vi "Dual_DM_Control_Main_V4.vi"() -> ()   [LabVIEW 2014]
uses:
  Controls/MirrorModes.ctl
  Controls/Standard Action.ctl
  <vilib>/Analysis/baseanly.llb/Mean (DBL).vi
  <vilib>/Utility/file.llb/Write To Spreadsheet File (DBL).vi
  <vilib>/Utility/file.llb/Read From Spreadsheet File (DBL).vi
  <vilib>/Analysis/NI_AALBase.lvlib
panel:
  in  "Active Mirror":enum32{"Mirror 1", "Mirror 2"}(radio)
  in  "Clear Modes":bool
  in  "Mirror Modes":T1
  in  "Load Modes":bool
  in  "Save Modes":bool
  in  "Scan Modes":bool
  in  "Load Flat":bool
  in  "Apply Zero":bool
  in  "Load V Map":bool
  in  "Save V Map":bool
  in  "Apply Flat":bool
  in  "Center Bias":bool
  in  "Exit":bool
  out "Pixel Map (-1 to 1)":dbl[][](graph)
  # "Mode"
  # "Amount (nm)"
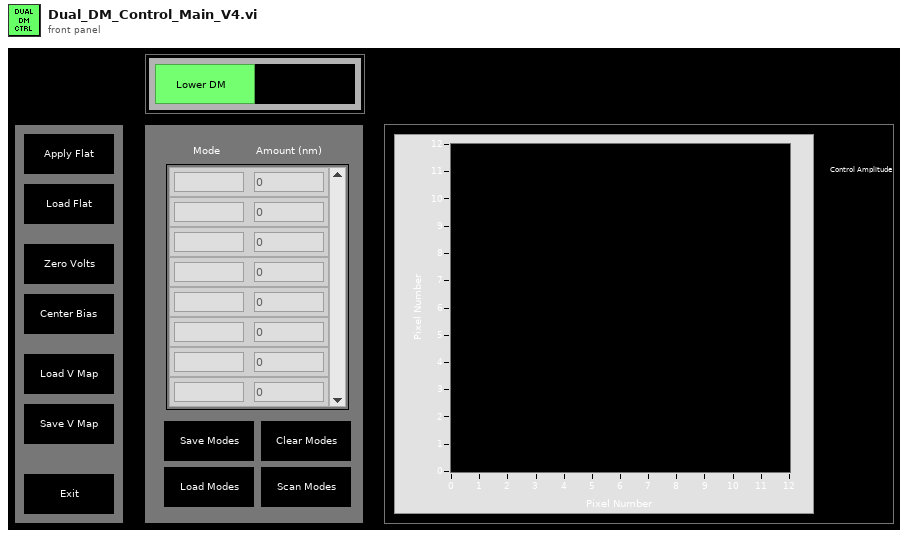
[diagram p1: front panel]
types:
  T1 = typedef "MirrorModes.ctl" = cluster{"Mode":string, "Amplitude":dbl}[]
  T2 = typedef "Standard Action.ctl" = enum16{"Read", "Write"}
  T3 = typedef "MirrorModes_DUAL.ctl" = cluster{"Mode":string, "Amplitude":dbl}[][]
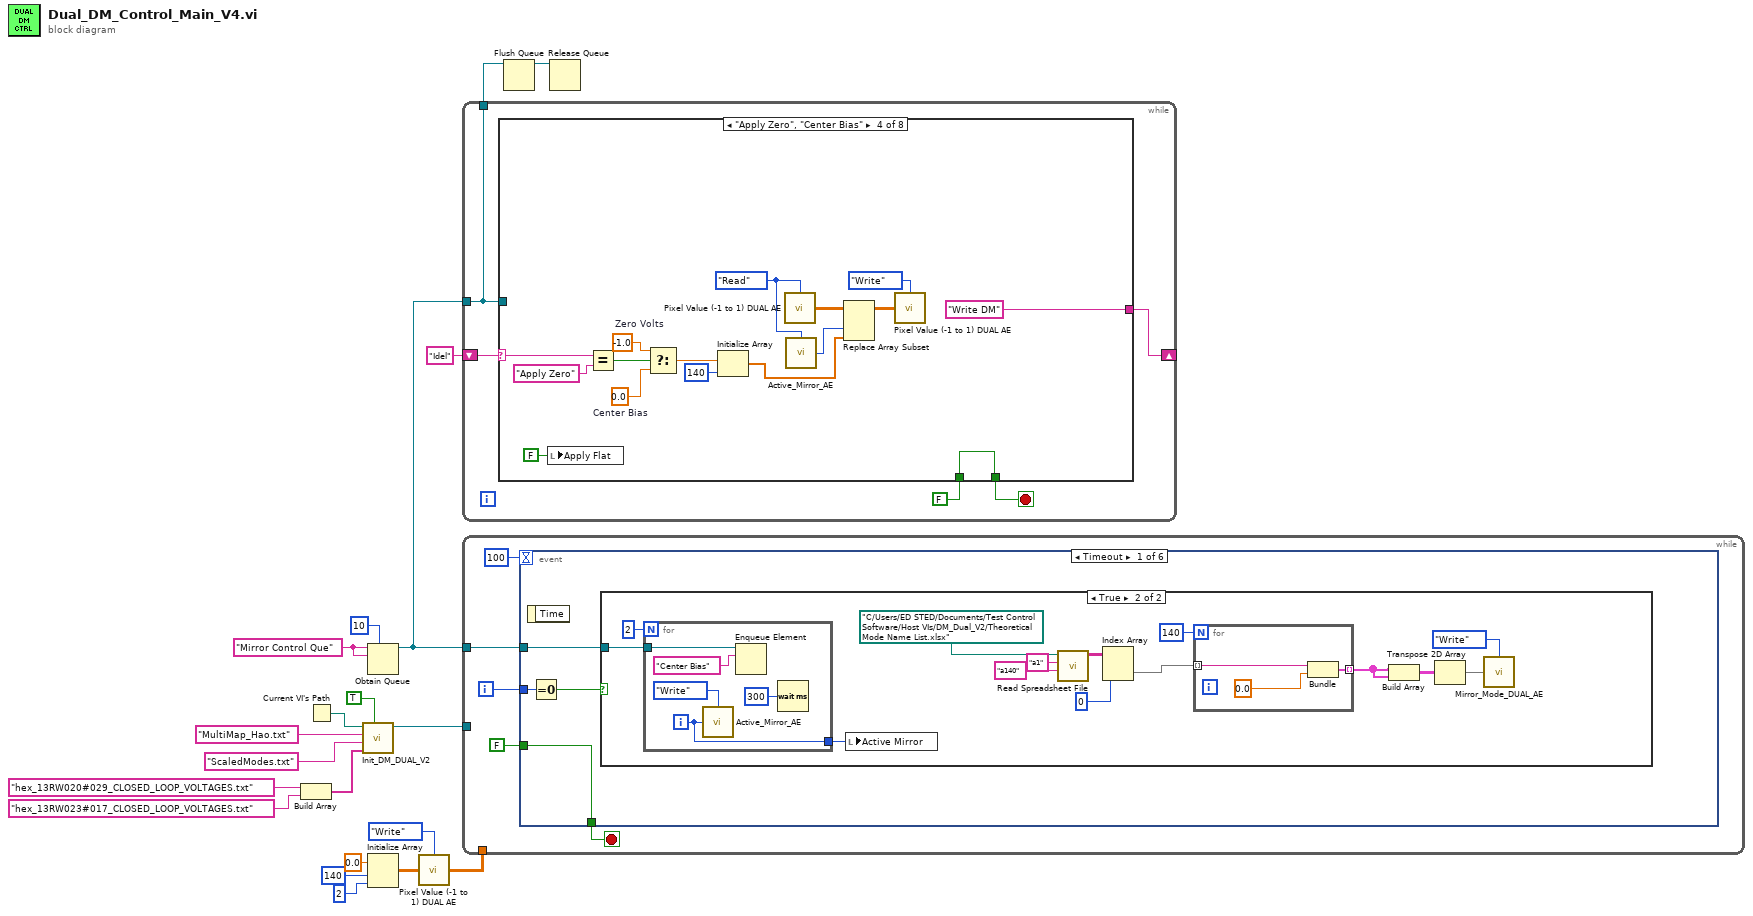
[diagram p0: block diagram]
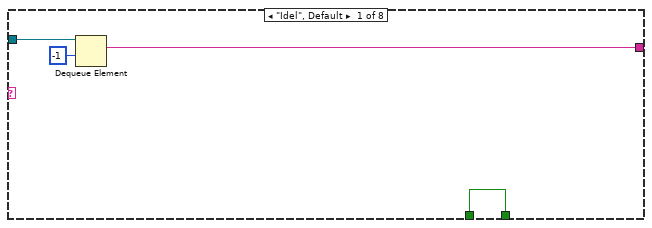
[diagram p2: hidden frame]
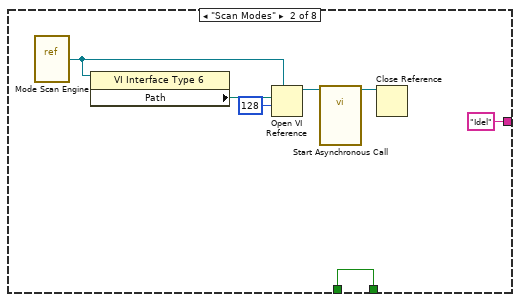
[diagram p3: hidden frame]
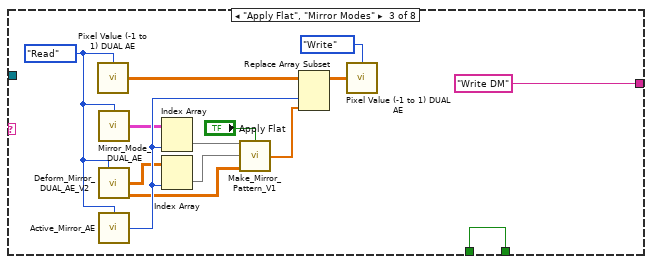
[diagram p4: hidden frame]
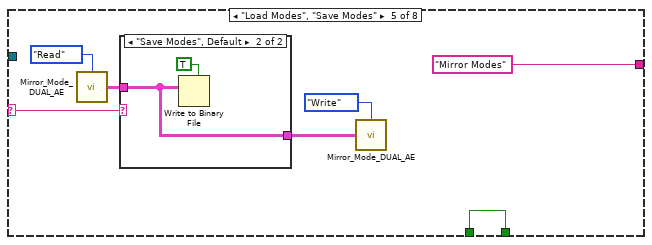
[diagram p5: hidden frame]
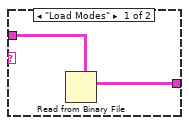
[diagram p6: hidden frame]
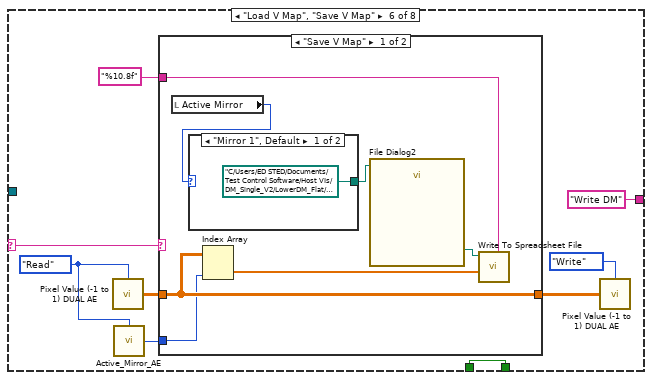
[diagram p7: hidden frame]
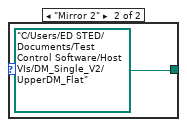
[diagram p8: hidden frame]
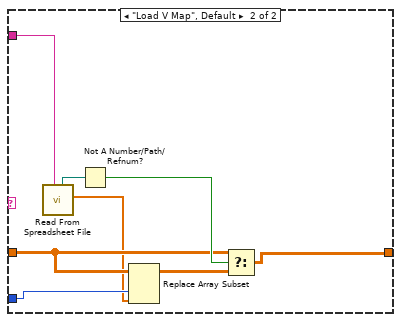
[diagram p9: hidden frame]
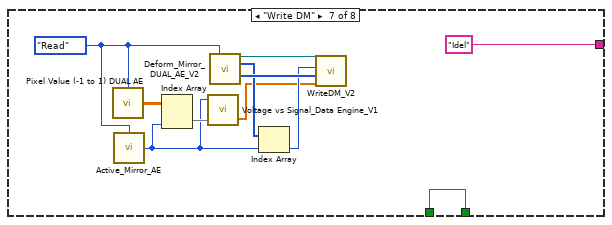
[diagram p10: hidden frame]
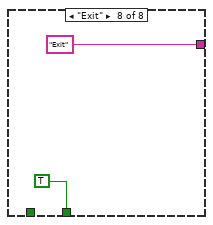
[diagram p11: hidden frame]
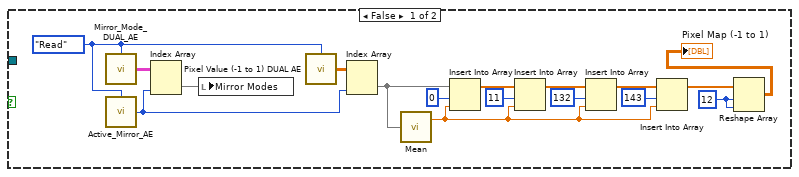
[diagram p12: hidden frame]
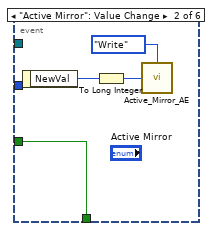
[diagram p13: hidden frame]
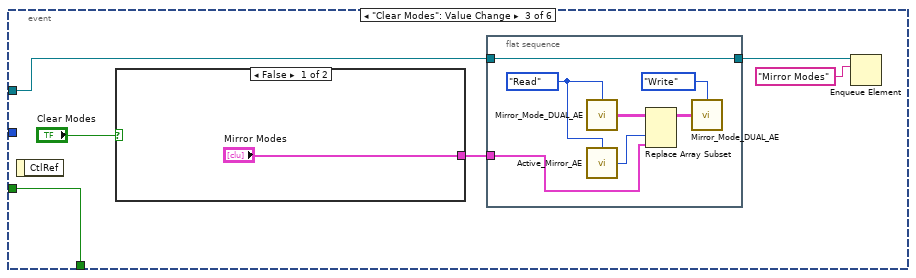
[diagram p14: hidden frame]
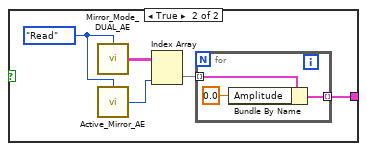
[diagram p15: hidden frame]
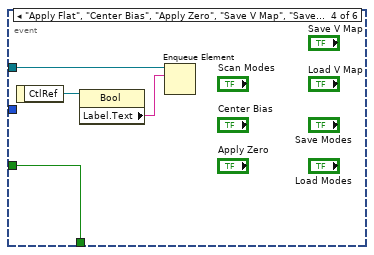
[diagram p16: hidden frame]
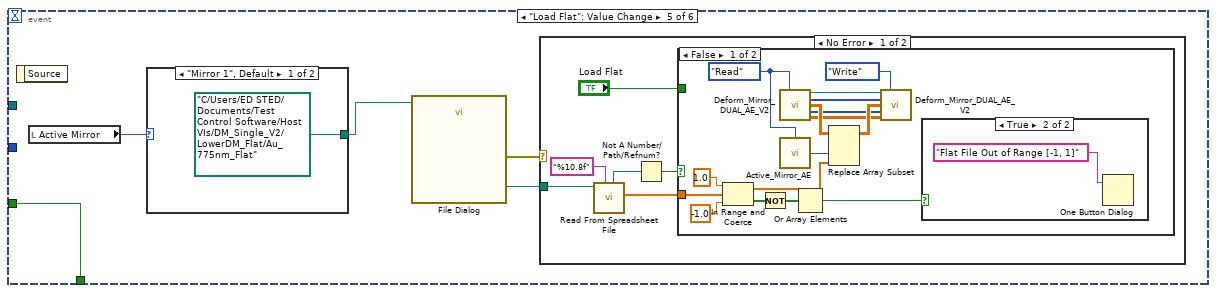
[diagram p17: hidden frame]
diagram:
  w20 = "Mirror Control Que" ("name (unnamed)")
  n1 = Build Array("hex_13RW020#029_CLOSED_LOOP_VOLTAGES.txt" ("name or relative path"), "hex_13RW023#017_CLOSED_LOOP_VOLTAGES.txt" ("name or relative path")) -> (w8:string[])
  n2 = Current VI's Path() -> (path=w12:path)
  n3 = call "Init_DM_DUAL_V2.vi"("BM Flat"=TRUE, "BM Flat File"=w8, "Mirror Modes File"="ScaledModes.txt" ("name or relative path"), "DM Mapping File"="MultiMap_Hao.txt" ("name or relative path"), "Base File Path"=w12) -> ("reference out"=w18:refnum<k7>)  [unwired: 6 in]
  n4 = Obtain Queue(max queue size (-1, unlimited)=10, name (unnamed)=w20, element data type=w20) -> (queue out=w14:refnum<queue>)  [unwired: 2 in, 2 out]
  n5 = Initialize Array(0.0 ("element"), 140 ("dimension size"), 2 ("dimension size")) -> (w4:dbl[][])
  n6 = call "Pixel Value (-1 to 1) DUAL AE.vi"("Action"=Standard_Action."Write", "Pixel Value (-1 to 1)"=w4) -> ("Pixel Value (-1 to 1) Out"=w2:dbl[][])  [unwired: 13 in]
  n7 = while {
    tunnel: w14 -> [w21]
    shift-right: [w25] -> _
    shift-left: "Idel" ("name (unnamed)") -> [w24]
    tunnel: [w21] -> w17
    stop <- w23 stop-if-true
    n8 = case shown="\"Apply Zero\", \"Center Bias\"" w24 {
      selector: w24 -> [_ _ _ w62 w69 w85 _ _]
      tunnel: w21 -> [w29 _ _ _ _ _ _ _]
      tunnel: [w27 "Idel" ("name (unnamed)") "Write DM" ("name (unnamed)") "Write DM" ("name (unnamed)") "Mirror Modes" ("name (unnamed)") "Write DM" ("name (unnamed)") "Idel" ("name (unnamed)") "Exit" ("name (unnamed)")] -> w25
      tunnel: [w26 w35 w49 w66 w73 w86 w114 TRUE] -> w23
      tunnel: FALSE -> [w26 w35 w49 w66 w73 w86 w114 _]
      frame "Idel", Default {
        n9 = Dequeue Element(queue=w29, timeout in ms (-1)=-1) -> (element=w27:string)  [unwired: 1 in, 3 out]
      }
      frame "Scan Modes" {
        n10 = vi-ref "Mode Scan Engine.vi"() -> (w30:refnum<vi>)
        n11 = property class="VI Interface Type 6"(reference=w30) -> ("Path"=w31:path)  [unwired: 1 in, 2 out]
        n12 = Open VI Reference(type specifier VI Refnum (for type only)=w30, vi path=w31, options=128) -> (vi reference=w33:refnum<vi>)  [unwired: 3 in, 1 out]
        n13 = call-by-ref "Start Asynchronous Call"(reference=w33) -> (reference out=w34:refnum<vi>)  [unwired: 3 in, 1 out]
        n14 = Close Reference(reference=w34) -> ()  [unwired: 1 in, 1 out]
      }
      frame "Apply Flat", "Mirror Modes" {
        w44 = Standard_Action."Read" ("Action")
        n15 = call "Pixel Value (-1 to 1) DUAL AE.vi"("Action"=w44) -> ("Pixel Value (-1 to 1) Out"=w45:dbl[][])  [unwired: 14 in]
        n16 = call "Mirror_Mode_DUAL_AE.vi"("Action"=w44) -> ("Mirror Modes Out"=w41:T3)  [unwired: 14 in]
        n17 = call "Deform_Mirror_DUAL_AE_V2.vi"("Action"=w44) -> ("Flat Files Out"=w39:dbl[][], "Mode Matrix Out"=w38:dbl[][])  [unwired: 10 in, 3 out]
        n18 = call "Active_Mirror_AE.vi"("Action"=w44) -> ("Active Mirror"=w47:i32)  [unwired: 14 in]
        n19 = Index Array(array=w41, index (col)=w47) -> (element=w42:cluster{"Mode":string, "Amplitude":dbl}[])  [unwired: 1 in]
        n20 = Index Array(array=w39, index (col)=w47) -> (element=w40:dbl[])  [unwired: 1 in]
        n21 = call "Make_Mirror_Pattern_V1.vi"("Mirror Modes In"=w42, "Flat On?"="Apply Flat", "Flat File In"=w40, "Mirror Modes Array"=w38) -> ("Pixel Value U (-1 to 1)"=w46:dbl[])  [unwired: 11 in]
        n22 = Replace Array Subset(array=w45, new element=w46, index (col)=w47) -> (w48:dbl[][])  [unwired: 1 in]
        n23 = call "Pixel Value (-1 to 1) DUAL AE.vi"("Action"=Standard_Action."Write", "Pixel Value (-1 to 1)"=w48) -> ()  [unwired: 13 in, 1 out]
      }
      frame "Apply Zero", "Center Bias" {
        w55 = Standard_Action."Read" ("Action")
        w58 = -1.0  # Zero Volts
        w60 = 0.0  # Center Bias
        n24 = local write "Apply Flat"(FALSE ("Apply Flat")) -> ()
        n25 = Equal?(x=w62, y="Apply Zero") -> (x = y?=w61:bool)
        n26 = Select(t=w58, s=w61, f=w60) -> (s? t:f=w59:dbl)
        n27 = Initialize Array(w59, 140 ("dimension size")) -> (w52:dbl[])
        n28 = call "Pixel Value (-1 to 1) DUAL AE.vi"("Action"=w55) -> ("Pixel Value (-1 to 1) Out"=w53:dbl[][])  [unwired: 14 in]
        n29 = call "Active_Mirror_AE.vi"("Action"=w55) -> ("Active Mirror"=w54:i32)  [unwired: 14 in]
        n30 = Replace Array Subset(array=w53, new element=w52, index (col)=w54) -> (w56:dbl[][])  [unwired: 1 in]
        n31 = call "Pixel Value (-1 to 1) DUAL AE.vi"("Action"=Standard_Action."Write", "Pixel Value (-1 to 1)"=w56) -> ()  [unwired: 13 in, 1 out]
      }
      frame "Load Modes", "Save Modes" {
        n32 = call "Mirror_Mode_DUAL_AE.vi"("Action"=Standard_Action."Read") -> ("Mirror Modes Out"=w68:T3)  [unwired: 14 in]
        n33 = case shown="\"Save Modes\", Default" w69 {
          tunnel: w68 -> [w75 w76]
          tunnel: [w74 w76] -> w67
          frame "Load Modes" {
            n34 = Read from Binary File(5:w75) -> (2:w74:T3)  [unwired: 5 in, 3 out]
          }
          frame "Save Modes", Default {
            n35 = Write to Binary File(data=w76, 5:TRUE ("prepend array or string size? (T)")) -> ()  [unwired: 4 in, 3 out]
          }
        }
        n36 = call "Mirror_Mode_DUAL_AE.vi"("Action"=Standard_Action."Write", "Mirror Modes In"=w67) -> ()  [unwired: 13 in, 1 out]
      }
      frame "Load V Map", "Save V Map" {
        w79 = Standard_Action."Read" ("Action")
        n37 = call "Pixel Value (-1 to 1) DUAL AE.vi"("Action"=w79) -> ("Pixel Value (-1 to 1) Out"=w83:dbl[][])  [unwired: 14 in]
        n38 = call "Active_Mirror_AE.vi"("Action"=w79) -> ("Active Mirror"=w78:i32)  [unwired: 14 in]
        n39 = case shown="\"Save V Map\"" w85 {
          tunnel: w83 -> [w92 w99]
          tunnel: "%10.8f" -> [w93 w103]
          tunnel: [w92 w100] -> w80
          tunnel: w78 -> [w90 w98]
          frame "Save V Map" {
            n40 = local read "Active Mirror"() -> (w88:enum32{"Mirror 1", "Mirror 2"})
            n41 = case shown="\"Mirror 1\", Default" w88 {
              tunnel: [path "C:/Users/ED STED/Documents/Test Control Software/Host VIs/DM_Single_V2/LowerDM_Flat/Au_775nm_Flat" path "C:/Users/ED STED/Documents/Test Control Software/Host VIs/DM_Single_V2/UpperDM_Flat"] -> w87
              frame "Mirror 1", Default {
              }
              frame "Mirror 2" {
              }
            }
            n42 = Index Array(array=w92, index (col)=w90) -> (element=w91:dbl[])  [unwired: 1 in]
            n43 = call "File Dialog2"("start path"=w87) -> ("selected path"=w89:path)  [unwired: 11 in, 3 out]
            n44 = call-poly <vilib>:"Write To Spreadsheet File.vi"("format (%.3f)"=w93, "1D data"=w91, "file path (dialog if empty)"=w89) -> ()  [unwired: 5 in, 1 out]
          }
          frame "Load V Map", Default {
            n45 = call-poly <vilib>:"Read From Spreadsheet File.vi"("format (%.3f)"=w103) -> ("first row"=w97:dbl[], "new file path (Not A Path if cancelled)"=w102:path)  [unwired: 6 in, 3 out]
            n46 = Not A Number/Path/Refnum?(number/path/refnum=w102) -> (NaN/Path/Refnum?=w101:bool)
            n47 = Replace Array Subset(array=w99, new element=w97, index (col)=w98) -> (w96:dbl[][])  [unwired: 1 in]
            n48 = Select(t=w99, s=w101, f=w96) -> (s? t:f=w100:dbl[][])
          }
        }
        n49 = call "Pixel Value (-1 to 1) DUAL AE.vi"("Action"=Standard_Action."Write", "Pixel Value (-1 to 1)"=w80) -> ()  [unwired: 13 in, 1 out]
      }
      frame "Write DM" {
        w109 = Standard_Action."Read" ("Action")
        n50 = call "Pixel Value (-1 to 1) DUAL AE.vi"("Action"=w109) -> ("Pixel Value (-1 to 1) Out"=w110:dbl[][])  [unwired: 14 in]
        n51 = call "Active_Mirror_AE.vi"("Action"=w109) -> ("Active Mirror"=w104:i32)  [unwired: 14 in]
        n52 = Index Array(array=w110, index (col)=w104) -> (element=w105:dbl[])  [unwired: 1 in]
        n53 = call "Voltage vs Signal_Data Engine_V1.vi"("Control Signal In (-1~1)"=w105, "DM #"=w104) -> ("Voltage Out (0~Max. Vol.)"=w106:dbl[])  [unwired: 1 in, 1 out]
        n54 = call "Deform_Mirror_DUAL_AE_V2.vi"("Action"=w109) -> ("Refnum Out"=w112:refnum<k7>, "IDs Out"=w108:i32[], "Multi Map Data Out"=w111:i32[])  [unwired: 10 in, 2 out]
        n55 = Index Array(array=w108, index=w104) -> (element=w107:i32)
        n56 = call "WriteDM_V2.vi"("reference in"=w112, "nDevId"=w107, "MultiDM  Mapping"=w111, "Voltage Array in"=w106) -> ()  [unwired: 2 in, 2 out]
      }
      frame "Exit" {
      }
    }
  }
  n57 = while {
    tunnel: w14 -> [w117]
    tunnel: w18 -> [_]
    tunnel: w2 -> [_]
    i -> [w118]
    stop <- w121 stop-if-true
    n58 = event shown="[0] Timeout" {
      selector: _ -> [_ _ _ _ _ _]
      dyn-events: _ -> [_ _ _ _ _ _]
      timeout: 100 -> [_ _ _ _ _ _]
      tunnel: [w125 w168 w174 w194 w199 w236] -> w121
      tunnel: FALSE -> [w125 w168 w174 w194 w199 _]
      tunnel: w118 -> [w124 _ _ _ _ _]
      tunnel: w117 -> [w122 _ w173 w193 _ w234]
      event Timeout {
        n59 = event-data() -> ()  [unwired: 1 in, 1 out]
        n60 = Equal To 0?(x=w124) -> (x = 0?=w123:bool)
        n61 = case shown="True" w123 {
          tunnel: w122 -> [_ w156]
          frame False {
            w138 = 12 ("dimension size")
            w139 = Standard_Action."Read" ("Action")
            n62 = call "Mirror_Mode_DUAL_AE.vi"("Action"=w139) -> ("Mirror Modes Out"=w126:T3)  [unwired: 14 in]
            n63 = call "Active_Mirror_AE.vi"("Action"=w139) -> ("Active Mirror"=w141:i32)  [unwired: 14 in]
            n64 = Index Array(array=w126, index (col)=w141) -> (element=w127:cluster{"Mode":string, "Amplitude":dbl}[])  [unwired: 1 in]
            n65 = local write "Mirror Modes"(w127) -> ()
            n66 = call "Pixel Value (-1 to 1) DUAL AE.vi"("Action"=w139) -> ("Pixel Value (-1 to 1) Out"=w140:dbl[][])  [unwired: 14 in]
            n67 = Index Array(array=w140, index (col)=w141) -> (element=w142:dbl[])  [unwired: 1 in]
            n68 = call-poly <vilib>:"Mean.vi"("X"=w142) -> ("mean"=w136:dbl)  [unwired: 1 out]
            n69 = Insert Into Array(array=w142, index=0, new element=w136) -> (w131:dbl[])
            n70 = Insert Into Array(array=w131, index=11, new element=w136) -> (w133:dbl[])
            n71 = Insert Into Array(array=w133, index=132, new element=w136) -> (w135:dbl[])
            n72 = Insert Into Array(array=w135, index=143, new element=w136) -> (w128:dbl[])
            n73 = Reshape Array(w128, w138, w138) -> (→"Pixel Map (-1 to 1)":dbl[][])
          }
          frame True {
            n74 = for {
              N: 2 -> [_]
              tunnel: w156 -> [w161]
              tunnel: [w157] -> w150
              i -> [w157]
              n75 = call "Active_Mirror_AE.vi"("Action"=Standard_Action."Write", "Active Mirror In"=w157) -> ()  [unwired: 13 in, 1 out]
              n76 = Enqueue Element(queue=w161, element="Center Bias") -> ()  [unwired: 2 in, 3 out]
              n77 = Wait (ms)(milliseconds to wait=u32 300) -> ()  [unwired: 1 out]
            }
            n78 = local write "Active Mirror"(w150) -> ()
            n79 = call "Read Spreadsheet File.vi"("End cell"="a140", "Start Cell"="a1", "path"=path "C:/Users/ED STED/Documents/Test Control Software/Host VIs/DM_Dual_V2/Theoretical Mode Name List.xlsx") -> ("Array"=w145:string[][])  [unwired: 7 in, 1 out]
            n80 = Index Array(array=w145, index (col)=0 ("disabled index (col)")) -> (element=w143:string[])  [unwired: 1 in]
            n81 = for {
              N: 140 -> [_]
              tunnel: [w163] -> w153 mode=indexing
              tunnel: w143 -> [w162] mode=indexing
              n82 = Bundle(w162, 0.0) -> (w163:cluster{string, dbl})  [unwired: 1 in]
            }
            n83 = Build Array(w153, w153) -> (w151:cluster{string, dbl}[][])
            n84 = Transpose 2D Array(2D array=w151) -> (transposed array=w146:cluster{string, dbl}[][])
            n85 = call "Mirror_Mode_DUAL_AE.vi"("Action"=Standard_Action."Write", "Mirror Modes In"=w146) -> ()  [unwired: 13 in, 1 out]
          }
        }
      }
      event "Active Mirror": Value Change {
        n86 = event-data() -> ("NewVal"=w167:enum32{"Mirror 1", "Mirror 2"})  [unwired: 1 in]
        n87 = To Long Integer(number=w167) -> (32bit integer=w166:i32)
        n88 = call "Active_Mirror_AE.vi"("Action"=Standard_Action."Write", "Active Mirror In"=w166) -> ()  [unwired: 13 in, 1 out]
      }
      event "Clear Modes": Value Change {
        n89 = event-data() -> ()  [unwired: 1 in, 1 out]
        n90 = case shown="False" "Clear Modes" {
          tunnel: ["Mirror Modes" w176] -> w169
          frame False {
          }
          frame True {
            w179 = Standard_Action."Read" ("Action")
            n91 = call "Mirror_Mode_DUAL_AE.vi"("Action"=w179) -> ("Mirror Modes Out"=w178:T3)  [unwired: 14 in]
            n92 = call "Active_Mirror_AE.vi"("Action"=w179) -> ("Active Mirror"=w180:i32)  [unwired: 14 in]
            n93 = Index Array(array=w178, index (col)=w180) -> (element=w177:cluster{"Mode":string, "Amplitude":dbl}[])  [unwired: 1 in]
            n94 = for {
              tunnel: w177 -> [w183] mode=indexing
              tunnel: [w181] -> w176 mode=indexing
              n95 = Bundle By Name(cluster=w183, "Amplitude"=0.0) -> (w181:cluster{"Mode":string, "Amplitude":dbl})
            }
          }
        }
        n96 = flat-sequence {
          tunnel: w169 -> [w184]
          tunnel: w173 -> [w190]
          tunnel: [w190] -> w171
          frame #0 {
            w187 = Standard_Action."Read" ("Action")
            n97 = call "Mirror_Mode_DUAL_AE.vi"("Action"=w187) -> ("Mirror Modes Out"=w186:T3)  [unwired: 14 in]
            n98 = call "Active_Mirror_AE.vi"("Action"=w187) -> ("Active Mirror"=w188:i32)  [unwired: 14 in]
            n99 = Replace Array Subset(array=w186, new element=w184, index (col)=w188) -> (w189:T3)  [unwired: 1 in]
            n100 = call "Mirror_Mode_DUAL_AE.vi"("Action"=Standard_Action."Write", "Mirror Modes In"=w189) -> ()  [unwired: 13 in, 1 out]
          }
        }
        n101 = Enqueue Element(queue=w171, element="Mirror Modes") -> ()  [unwired: 2 in, 3 out]
      }
      event "Apply Flat", "Center Bias", "Apply Zero", "Save V Map", "Save Modes", "Load Modes", "Load V Map", "Scan Modes": Value Change {
        n102 = event-data() -> ("CtlRef"=w192:refnum<vi>)  [unwired: 1 in]
        n103 = property class="Bool"(reference=w192) -> ("Label.Text"=w191:string)  [unwired: 1 in, 2 out]
        n104 = Enqueue Element(queue=w193, element=w191) -> ()  [unwired: 2 in, 3 out]
      }
      event "Load Flat": Value Change {
        n105 = event-data() -> ()  [unwired: 1 in, 1 out]
        n106 = local read "Active Mirror"() -> (w197:enum32{"Mirror 1", "Mirror 2"})
        n107 = case shown="\"Mirror 1\", Default" w197 {
          tunnel: [path "C:/Users/ED STED/Documents/Test Control Software/Host VIs/DM_Single_V2/LowerDM_Flat/Au_775nm_Flat" path "C:/Users/ED STED/Documents/Test Control Software/Host VIs/DM_Single_V2/UpperDM_Flat"] -> w196
          frame "Mirror 1", Default {
          }
          frame "Mirror 2" {
          }
        }
        n108 = call "File Dialog"("start path"=w196) -> ("selected path"=w198:path, "error out"=w195:errorcluster)  [unwired: 11 in, 2 out]
        n109 = case shown="No Error" w195 {
          tunnel: w198 -> [w200 _]
          frame No Error {
            n110 = call-poly <vilib>:"Read From Spreadsheet File.vi"("format (%.3f)"="%10.8f", "file path (dialog if empty)"=w200) -> ("first row"=w202:dbl[], "new file path (Not A Path if cancelled)"=w204:path)  [unwired: 5 in, 3 out]
            n111 = Not A Number/Path/Refnum?(number/path/refnum=w204) -> (NaN/Path/Refnum?=w203:bool)
            n112 = case shown="False" w203 {
              tunnel: w202 -> [w221 _]
              tunnel: "Load Flat" -> [_ _]
              frame False {
                w212 = Standard_Action."Read" ("Action")
                n113 = In Range and Coerce(upper limit=1.0, x=w221, lower limit=-1.0) -> (coerced(x)=w206:dbl[], In Range?=w218:bool[])
                n114 = Not(x=w218) -> (.not. x?=w217:bool[])
                n115 = call "Deform_Mirror_DUAL_AE_V2.vi"("Action"=w212) -> ("Refnum Out"=w207:refnum<k7>, "IDs Out"=w208:i32[], "Flat Files Out"=w213:dbl[][], "Multi Map Data Out"=w209:i32[], "Mode Matrix Out"=w210:dbl[][])  [unwired: 10 in]
                n116 = call "Active_Mirror_AE.vi"("Action"=w212) -> ("Active Mirror"=w215:i32)  [unwired: 14 in]
                n117 = Or Array Elements(Boolean array=w217) -> (logical OR=w216:bool)
                n118 = Replace Array Subset(array=w213, new element=w206, index (col)=w215) -> (w214:dbl[][])  [unwired: 1 in]
                n119 = call "Deform_Mirror_DUAL_AE_V2.vi"("Refnum In"=w207, "Action"=Standard_Action."Write", "IDs In"=w208, "Flat Files In"=w214, "Multi Map Data In"=w209, "Mode Matrix"=w210) -> ()  [unwired: 5 in, 5 out]
                n120 = case shown="True" w216 {
                  frame False {
                  }
                  frame True {
                    n121 = One Button Dialog(message="Flat File Out of Range [-1, 1]") -> ()  [unwired: 1 in, 1 out]
                  }
                }
              }
              frame True {
              }
            }
          }
          frame Error {
          }
        }
      }
      event "Exit": Value Change {
        n122 = event-data() -> ("NewVal"=w236:bool)  [unwired: 1 in]
        n123 = for {
          N: 2 -> [_]
          tunnel: w234 -> [w242]
          tunnel: [w237] -> w225
          i -> [w238]
          n124 = call "Active_Mirror_AE.vi"("Action"=Standard_Action."Write", "Active Mirror In"=w238) -> ()  [unwired: 13 in, 1 out]
          n125 = Enqueue Element(queue=w242, element="Apply Zero") -> (queue out=w237:refnum<queue>)  [unwired: 2 in, 2 out]
          n126 = Wait (ms)(milliseconds to wait=u32 300) -> ()  [unwired: 1 out]
        }
        n127 = Enqueue Element(queue=w225, element="Exit") -> (error out=w229:errorcluster)  [unwired: 2 in, 2 out]
        n128 = call "Deform_Mirror_DUAL_AE_V2.vi"("Action"=Standard_Action."Read") -> ("Refnum Out"=w232:refnum<k7>, "IDs Out"=w227:i32[])  [unwired: 10 in, 3 out]
        n129 = call "ConfigDM.vi"("High Voltage"=FALSE, "error in (no error)"=w229, "Dev IDs"=w227, "Automation Refnum in"=w232) -> ("error out"=w228:errorcluster, "Automation Refnum out"=w231:refnum<k7>)  [unwired: 6 in]
        n130 = Close Reference(reference=w231, error in (no error)=w228) -> ()  [unwired: 1 out]
      }
    }
  }
  n131 = Flush Queue(queue=w17) -> (queue out=w16:refnum<queue>)  [unwired: 1 in, 2 out]
  n132 = Release Queue(queue=w16) -> ()  [unwired: 2 in, 3 out]
